vi "addDelayTicks.vi"(8 "error in (no error)":errorcluster, 10 "Ticks":u16, 11 "Subnet in":refnum<class "ISubnet.lvclass">) -> (0 "error out":errorcluster, 3 "Subnet out":refnum<class "ISubnet.lvclass">)   [LabVIEW 2015, in "ISubnet.lvclass"]
uses:
  ISubnet.lvclass
  ISubnet.lvclass/ISubnet.ctl
  Common_RT_Modbus/IModbus/IModbus.lvclass
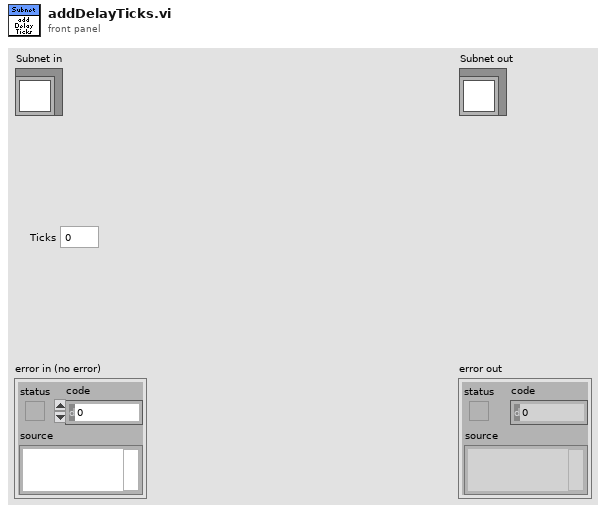
[diagram p1: front panel]
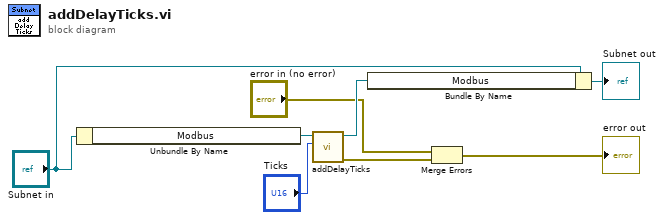
[diagram p0: block diagram]
diagram:
  n1 = Unbundle By Name("Subnet in") -> ("Modbus"=w6:refnum<class "IModbus.lvclass">)
  n2 = call-dynamic "addDelayTicks.vi"("Ticks"="Ticks", "IModbus in"=w6) -> ("error out"=w3:errorcluster, "IModbus out"=w5:refnum<class "IModbus.lvclass">)  [unwired: 8 in]
  n3 = Bundle By Name(cluster="Subnet in", "Modbus"=w5) -> (→"Subnet out":refnum<class "ISubnet.lvclass">)
  n4 = Merge Errors("error in (no error)", w3) -> (→"error out":errorcluster)
